vi "Create castle restricting move.vi"(4 "Restrict queen side (F)":bool, 6 "Restrict king side (F)":bool, 8 "error in (no error)":errorcluster, 9 "Destination":T1={"File"=enum."d", "Rank"=enum."4"}, 10 "Source":T1={"File"=enum."d", "Rank"=enum."4"}) -> (0 "error out":errorcluster, 3 "CastleRestricting out":refnum<class "CastleRestricting.lvclass">)   [LabVIEW 2016, in "Chesslib.lvlib" / "CastleRestricting.lvclass"]
uses:
  CastleRestricting.lvclass
  C:/Users/GRTaggJ/Documents/Projects/chesslib/Moves/Move/Move.lvclass
  typedef/Square.ctl
  typedef/File.ctl
  typedef/Rank.ctl
  CastleRestricting.lvclass/CastleRestricting.ctl
  Move/Move.lvclass
  Chesslib.lvlib
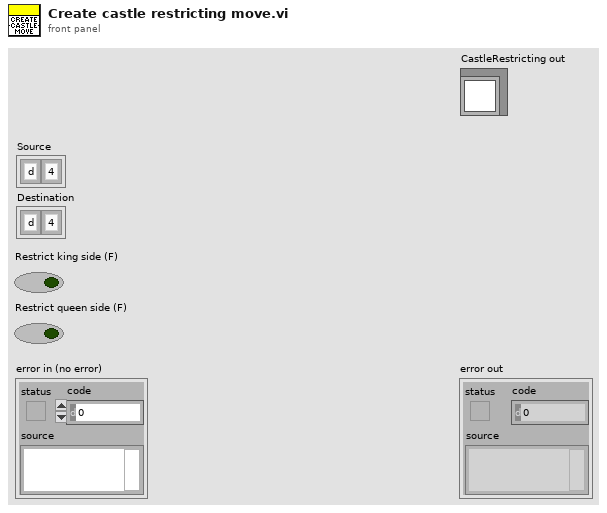
[diagram p1: front panel]
types:
  T1 = typedef "Chesslib.lvlib/Square.ctl" = cluster{"File":T2, "Rank":T3}
  T2 = typedef "Chesslib.lvlib/File.ctl" = enum8{"a", "b", "c", "d", "e", "f", "g", "h"}
  T3 = typedef "Chesslib.lvlib/Rank.ctl" = enum8{"1", "2", "3", "4", "5", "6", "7", "8"}
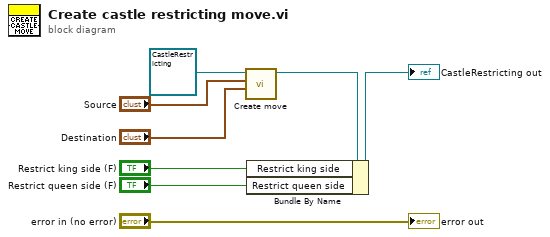
[diagram p0: block diagram]
diagram:
  n1 = call "Create move.vi"("Destination"="Destination", "Source"="Source", "Move in"=refnum<class "CastleRestricting.lvclass"> refnum ("CastleRestricting in")) -> ("Move out"=w6:refnum<class "CastleRestricting.lvclass">)  [unwired: 8 in]
  n2 = Bundle By Name(cluster=w6, "Restrict king side"="Restrict king side (F)", "Restrict queen side"="Restrict queen side (F)") -> (→"CastleRestricting out":refnum<class "CastleRestricting.lvclass">)
  "error out" <- "error in (no error)"
